vi "InitializeLogging.vi"(8 "error in (no error)":errorcluster, 11 "Column Names":string[](array[string])) -> (0 "error out":errorcluster, 3 "Headers String":string)   [LabVIEW 2017]
uses:
  LogOperation.ctl
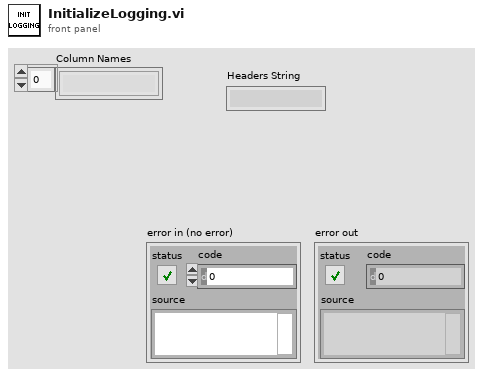
[diagram p1: front panel]
types:
  T1 = typedef "LogOperation.ctl" = enum16{"Set", "Get All", "Init"}
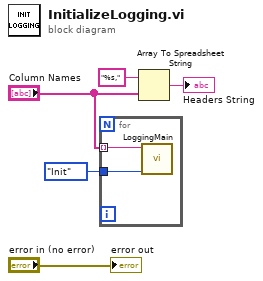
[diagram p0: block diagram]
diagram:
  n1 = for {
    tunnel: "Column Names" -> [w7] mode=indexing
    tunnel: LogOperation."Init" ("Operation") -> [w6]
    n2 = call "LoggingMain.vi"("Operation"=w6, "Name"=w7) -> ()  [unwired: 9 in, 1 out]
  }
  n3 = Array To Spreadsheet String(array="Column Names", 3:"%s," ("format string")) -> (spreadsheet string=→"Headers String":string)  [unwired: 1 in]
  "error out" <- "error in (no error)"
